vi "Write Parameters (array).vi"(8 "error in (no error)":errorcluster, 10 "Parameters":string[][](array[string]), 11 "Run Instance in":refnum<class "Run Instance.lvclass">) -> (0 "error out":errorcluster, 3 "Run Instance out":refnum<class "Run Instance.lvclass">)   [LabVIEW 2020, in "Run Utilities.lvlib" / "Run Instance.lvclass"]
uses:
  Run Instance.lvclass
  Run Instance.lvclass/Run Instance.ctl
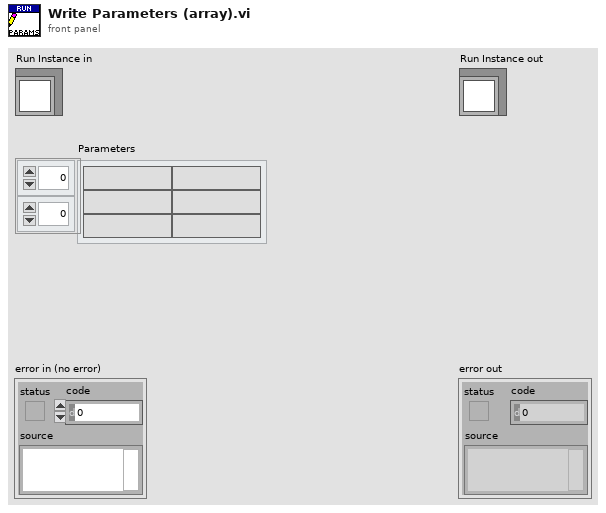
[diagram p1: front panel]
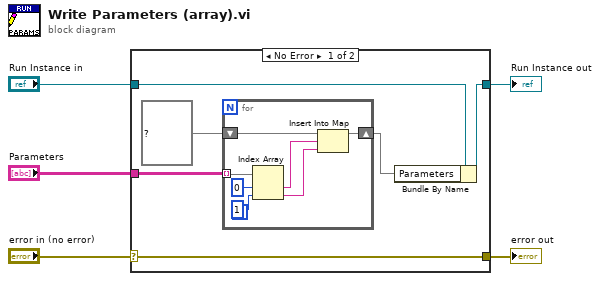
[diagram p0: block diagram]
diagram:
  n1 = case shown="No Error" "error in (no error)" {
    selector: "error in (no error)" -> [w11 w19]
    tunnel: [w11 w19] -> w4
    tunnel: [w9 w20] -> w2
    tunnel: "Run Instance in" -> [w10 w20]
    tunnel: "Parameters" -> [w8 _]
    frame No Error {
      n2 = for {
        tunnel: w8 -> [w18] mode=indexing
        shift-right: [w12] -> w6
        shift-left: map{string, string} {} ("Parameters") -> [w13]
        n3 = Index Array(array=w18, index #1=0 ("index"), index #2=1 ("index")) -> (element #1=w15:string, element #2=w14:string)
        n4 = Insert Into Map(map in=w13, key=w15, value=w14) -> (map out=w12:map{string, string})  [unwired: 2 out]
      }
      n5 = Bundle By Name(cluster=w10, "Parameters"=w6) -> (w9:refnum<class "Run Instance.lvclass">)
    }
    frame Error {
    }
  }
  "error out" <- w4
  "Run Instance out" <- w2
